vi "Motion Profile Generator-Demo.vi"(0 "Max Speed (rotations/sec)":dbl=3.0, 5 "Max Acceleration (rotations/sec^2)":dbl=1.0, 7 "Max Jerk (rotations/sec^3)":dbl=1.0, 9 "Rotations to Travel":dbl=4.0, 11 "Motion Profile Control Frame Rate":dbl=10.0) -> (4 "Position rotations":dbl[](array[numeric]), 6 "velocity rotations/sec":dbl[](array[numeric]), 8 "acceleration rotations/sec^2":dbl[](array[numeric]), 10 "XY Graph":cluster{dbl[], dbl[]}[](graph))   [LabVIEW 2015]
panel:
  out "Final Position":dbl
  # "This VI uses the \"Copioli\" Method of Motion Profiling. For more information read this chief delphi thread: http://www.chiefdelphi.com/forums/showthread.php?t=98358&highlight=motion+profile"
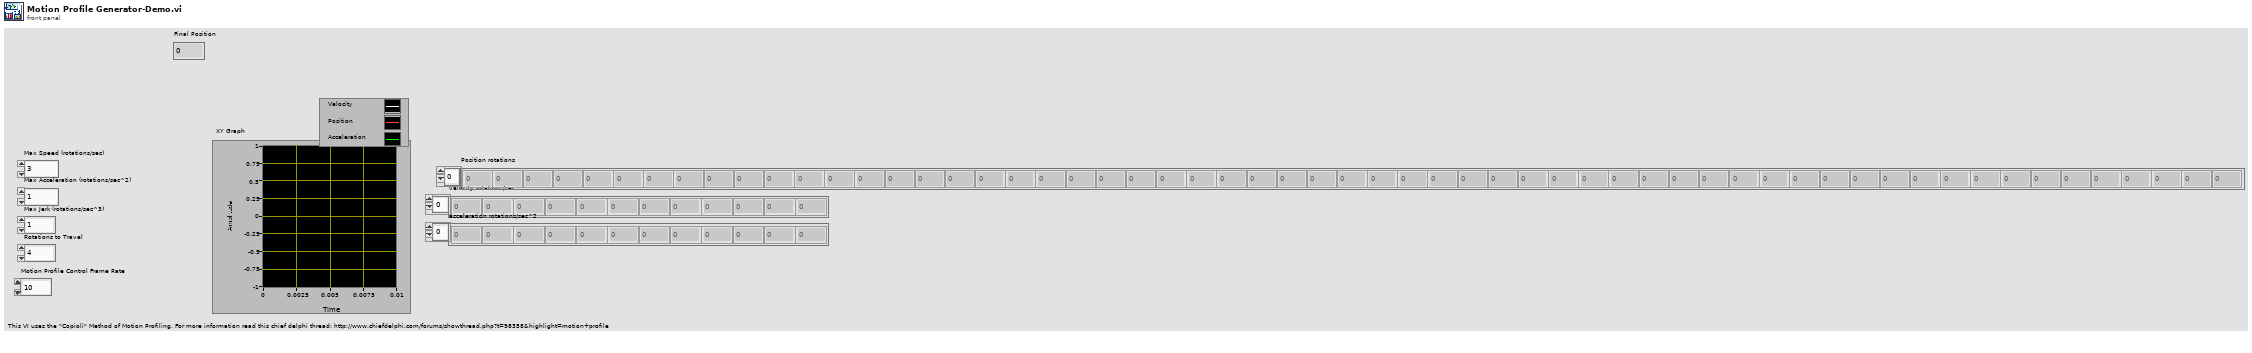
[diagram p1: front panel]
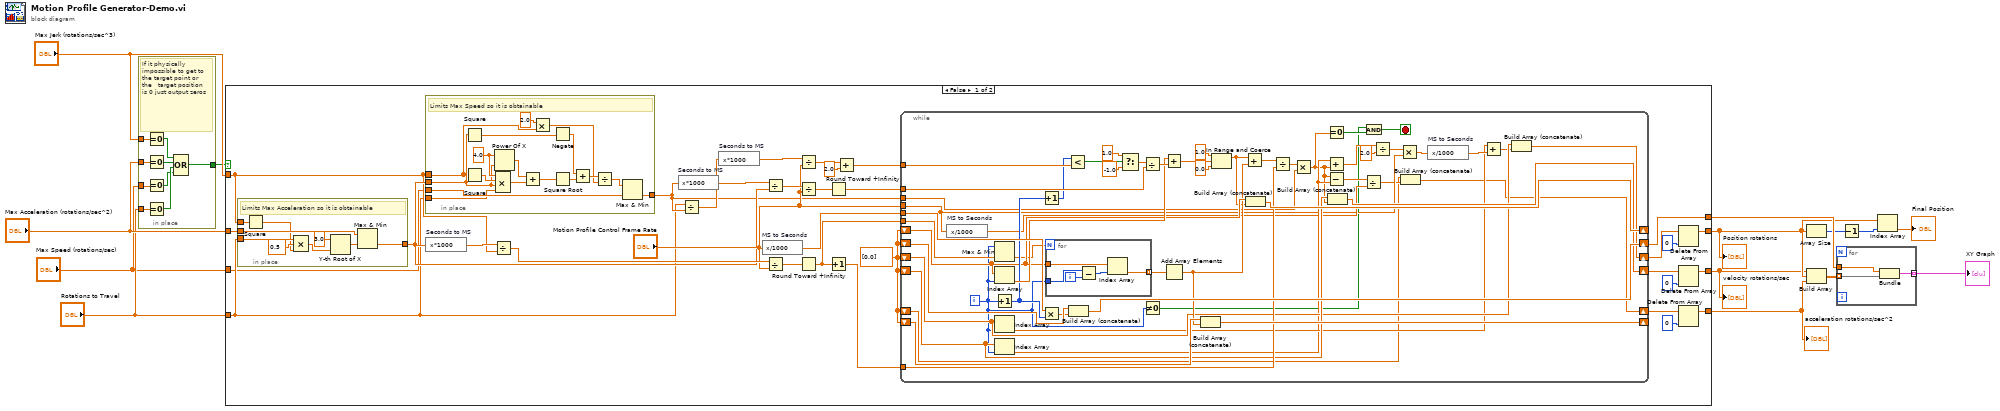
[diagram p0: block diagram]
diagram:
  n1 = in-place {
    in-place-border: "Max Jerk (rotations/sec^3)" -> [w23]
    in-place-border: "Max Acceleration (rotations/sec^2)" -> [w22]
    in-place-border: "Rotations to Travel" -> [w21]
    in-place-border: [w17] -> w2
    in-place-border: "Max Speed (rotations/sec)" -> [w15]
    # "If it physically impossible to get to the target point or the   target position is 0 just output zeros"
    n2 = Equal To 0?(x=w23) -> (x = 0?=w20:bool)
    n3 = Equal To 0?(x=w22) -> (x = 0?=w19:bool)
    n4 = Equal To 0?(x=w15) -> (x = 0?=w16:bool)
    n5 = Equal To 0?(x=w21) -> (x = 0?=w18:bool)
    n6 = Compound Arithmetic op=OR(w20, w19, w18, w16) -> (w17:bool)
  }
  n7 = case shown="False" w2 {
    tunnel: [w39 _] -> w13
    tunnel: [w33 _] -> w8
    tunnel: [w29 _] -> w7
    tunnel: [w28 _] -> w6
    tunnel: "Max Jerk (rotations/sec^3)" -> [w27 _]
    tunnel: "Max Acceleration (rotations/sec^2)" -> [w26 _]
    tunnel: "Rotations to Travel" -> [w25 _]
    tunnel: "Max Speed (rotations/sec)" -> [w24 _]
    frame False {
      w40 = dbl[] [0.0]
      n8 = in-place {
        in-place-border: w27 -> [w65]
        in-place-border: w26 -> [w63]
        in-place-border: [w62] -> w38
        in-place-border: w25 -> [w61]
        # "Limits Max Acceleration so it is obtainable"
        n9 = Square(x=w65) -> (x^2=w59:dbl)
        n10 = Compound Arithmetic op=MULTIPLY(w61, 0.5 ("value"), w59) -> (w58:dbl)
        n11 = Y-th Root of X(1:w58, 2:3.0 ("y")) -> (0:w64:dbl)
        n12 = Max & Min(x=w63, y=w64) -> (min(x,y)=w62:dbl)  [unwired: 1 out]
      }
      n13 = in-place {
        in-place-border: w24 -> [w82]
        in-place-border: [w69] -> w37
        in-place-border: w38 -> [w75]
        in-place-border: w25 -> [w74]
        in-place-border: w27 -> [w71]
        w78 = 4.0 ("x")
        # "Limits Max Speed so it is obtainable"
        n14 = Square(x=w75) -> (x^2=w81:dbl)
        n15 = Square(x=w71) -> (x^2=w77:dbl)
        n16 = Power Of X(1:w75, 2:w78) -> (0:w79:dbl)
        n17 = Compound Arithmetic op=MULTIPLY(w78, w77, w75, w74) -> (w76:dbl)
        n18 = Add(x=w79, y=w76) -> (x+y=w73:dbl)
        n19 = Multiply(x=2.0, y=w71) -> (x*y=w66:dbl)
        n20 = Negate(x=w81) -> (-x=w80:dbl)
        n21 = Square Root(x=w73) -> (sqrt(x)=w70:dbl)
        n22 = Add(x=w80, y=w70) -> (x+y=w68:dbl)
        n23 = Divide(x=w68, y=w66) -> (x/y=w67:dbl)
        n24 = Max & Min(x=w67, y=w82) -> (min(x,y)=w69:dbl)  [unwired: 1 out]
      }
      n25 = expression code="x*1000" "Seconds to MS"(w38) -> (w55:dbl)
      n26 = Divide(x=w55, y=w27) -> (x/y=w45:dbl)
      n27 = expression code="x*1000" "Seconds to MS"(w37) -> (w54:dbl)
      n28 = Divide(x=w25, y=w37) -> (x/y=w53:dbl)
      n29 = expression code="x*1000" "Seconds to MS"(w53) -> (w52:dbl)
      n30 = expression code="x/1000" "MS to Seconds"("Motion Profile Control Frame Rate") -> (w56:dbl)
      n31 = Divide(x=w54, y=w38) -> (x/y=w48:dbl)
      n32 = Divide(x=w45, y="Motion Profile Control Frame Rate") -> (x/y=w44:dbl)
      n33 = Divide(x=w52, y="Motion Profile Control Frame Rate") -> (x/y=w51:dbl)
      n34 = Divide(x=w48, y="Motion Profile Control Frame Rate") -> (x/y=w47:dbl)
      n35 = Round Toward +Infinity(x=w44) -> (ceil(x): smallest int >= x=w43:dbl)
      n36 = Round Toward +Infinity(x=w47) -> (ceil(x): smallest int >= x=w46:dbl)
      n37 = Increment(x=w43) -> (x+1=w42:dbl)
      n38 = Add(x=w51, y=2.0) -> (x+y=w49:dbl)
      n39 = while {
        shift-right: [w134] -> w39
        shift-left: w40 -> [w135]
        tunnel: w56 -> [w133]
        tunnel: w49 -> [w131]
        shift-right: [w121] -> _
        shift-left: w40 -> [w120]
        tunnel: w46 -> [w126]
        tunnel: w43 -> [w118]
        shift-right: [w115] -> _
        shift-left: w40 -> [w116]
        tunnel: w42 -> [w112]
        tunnel: w37 -> [w110]
        shift-right: [w109] -> w32
        shift-left: w40 -> [w107]
        shift-right: [w108] -> w30
        shift-left: w40 -> [w101]
        tunnel: "Motion Profile Control Frame Rate" -> [w95]
        shift-right: [w93] -> w34
        shift-left: w40 -> [w92]
        i -> [w91]
        stop <- w87 stop-if-true
        n40 = expression code="x/1000" "MS to Seconds"(w95) -> (w96:dbl)
        n41 = Max & Min(x=w91, y=w118) -> (min(x,y)=w117:dbl)  [unwired: 1 out]
        n42 = Index Array(array=w120, index=w91) -> (element=w124:dbl)
        n43 = Increment(x=w91) -> (x+1=w122:i32)
        n44 = Index Array(array=w101, index=w91) -> (element=w100:dbl)
        n45 = Index Array(array=w107, index=w91) -> (element=w98:dbl)
        n46 = Increment(x=w122) -> (x+1=w123:i32)
        n47 = Multiply(x=w133, y=w122) -> (x*y=w132:dbl)
        n48 = for {
          N: w117 -> [_]
          tunnel: w91 -> [w139]
          tunnel: w120 -> [w137]
          tunnel: [w136] -> w119 mode=indexing
          i -> [w140]
          n49 = Subtract(x=w139, y=w140) -> (x-y=w138:i32)
          n50 = Index Array(array=w137, index=w138) -> (element=w136:dbl)
        }
        n51 = Less?(x=w123, y=w131) -> (x < y?=w130:bool)
        n52 = Build Array (concatenate)(w135, w132) -> (w134:dbl[])
        n53 = Select(t=1.0, s=w130, f=-1.0) -> (s? t:f=w127:dbl)
        n54 = Divide(x=w127, y=w126) -> (x/y=w125:dbl)
        n55 = Not Equal To 0?(x=w91) -> (x != 0?=w88:bool)
        n56 = Add(x=w124, y=w125) -> (x+y=w84:dbl)
        n57 = Add Array Elements(numeric array=w119) -> (sum=w114:dbl)
        n58 = Build Array (concatenate)(w116, w114) -> (w115:dbl[])
        n59 = In Range and Coerce(upper limit=1.0, x=w84, lower limit=0.0) -> (coerced(x)=w83:dbl)  [unwired: 1 out]
        n60 = Add(x=w83, y=w114) -> (x+y=w113:dbl)
        n61 = Build Array (concatenate)(w120, w83) -> (w121:dbl[])
        n62 = Divide(x=w113, y=w112) -> (x/y=w111:dbl)
        n63 = Multiply(x=w111, y=w110) -> (x*y=w90:dbl)
        n64 = Add(x=w98, y=w90) -> (x+y=w106:dbl)
        n65 = Subtract(x=w90, y=w98) -> (x-y=w97:dbl)
        n66 = Equal To 0?(x=w90) -> (x = 0?=w89:bool)
        n67 = Build Array (concatenate)(w107, w90) -> (w109:dbl[])
        n68 = Divide(x=w97, y=w96) -> (x/y=w94:dbl)
        n69 = And(x=w88, y=w89) -> (x .and. y?=w87:bool)
        n70 = Divide(x=w106, y=2.0) -> (x/y=w104:dbl)
        n71 = Multiply(x=w104, y=w95) -> (x*y=w103:dbl)
        n72 = Build Array (concatenate)(w92, w94) -> (w93:dbl[])
        n73 = expression code="x/1000" "MS to Seconds"(w103) -> (w102:dbl)
        n74 = Add(x=w100, y=w102) -> (x+y=w99:dbl)
        n75 = Build Array (concatenate)(w101, w99) -> (w108:dbl[])
      }
      n76 = Delete From Array(array=w30, index=0) -> (array with subset deleted=w29:dbl[])  [unwired: 1 in, 1 out]
      n77 = Delete From Array(array=w32, index=0) -> (array with subset deleted=w28:dbl[])  [unwired: 1 in, 1 out]
      n78 = Delete From Array(array=w34, index=0) -> (array with subset deleted=w33:dbl[])  [unwired: 1 in, 1 out]
    }
    frame True {
    }
  }
  "velocity rotations/sec" <- w6
  "Position rotations" <- w7
  "acceleration rotations/sec^2" <- w8
  n79 = Array Size(array=w7) -> (size(s)=w11:i32)
  n80 = Build Array(w6, w7, w8) -> (w14:dbl[][])
  n81 = for {
    tunnel: w14 -> [w143] mode=indexing
    tunnel: w13 -> [w142]
    tunnel: [w141] -> w12 mode=indexing
    n82 = Bundle(w142, w143) -> (w141:cluster{dbl[], dbl[]})  [unwired: 1 in]
  }
  "XY Graph" <- w12
  n83 = Decrement(x=w11) -> (x-1=w10:i32)
  n84 = Index Array(array=w7, index=w10) -> (element=→"Final Position":dbl)
